vi "Get Valid Properties.vi"(8 "error in (no error)":errorcluster, 11 "FM Sweep in":refnum<class "FM Sweep.lvclass">) -> (0 "error out":errorcluster, 2 "Properties":string[](array[string]), 3 "FM Sweep out":refnum<class "FM Sweep.lvclass">)   [LabVIEW 2020, in "FM Sweep.lvclass"]
uses:
  FM Sweep.lvclass
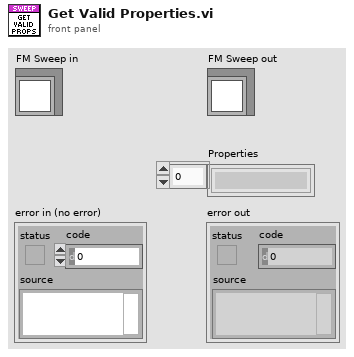
[diagram p1: front panel]
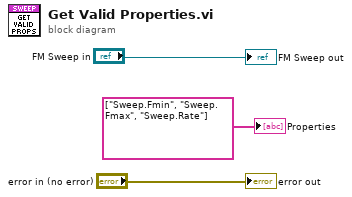
[diagram p0: block diagram]
diagram:
  "error out" <- "error in (no error)"
  "FM Sweep out" <- "FM Sweep in"
  "Properties" <- string[] ["Sweep.Fmin", "Sweep.Fmax", "Sweep.Rate"] ("Properties")
